vi "Init PWM Resources.vi"(8 "error in (no error)":errorcluster, 11 "Session in":refnum<class "Session.lvclass">) -> (0 "error out":errorcluster, 3 "Session out":refnum<class "Session.lvclass">)   [LabVIEW 2020, in "CTI.lvlib" / "Session.lvclass"]
uses:
  Session.lvclass
  GPIO Number.ctl
  PWM/PWM.lvclass
  Session.lvclass/Session.ctl
  CTI.lvlib
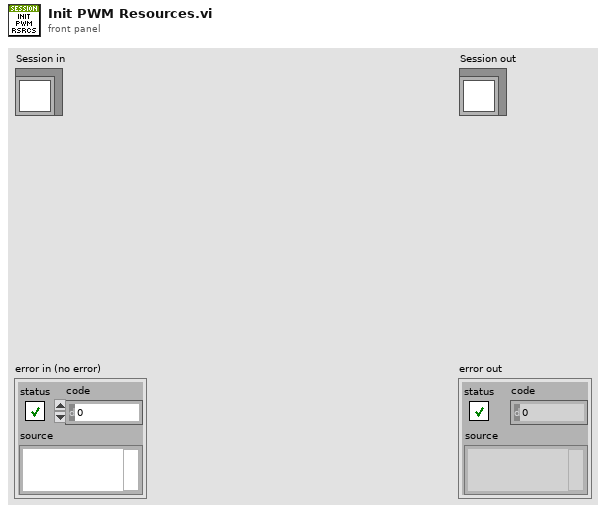
[diagram p1: front panel]
types:
  T1 = typedef "CTI.lvlib/GPIO Number.ctl" = i8
  T2 = typedef "CTI.lvlib/Session.lvclass/Resources.ctl" = cluster{"GPIO":map{T1, refnum<class "GPIO.lvclass">}, "AI":map{T3, refnum<class "AI.lvclass">}, "PWM":map{T1, refnum<class "PWM.lvclass">}, "UART":map{T4, refnum<class "UART.lvclass">}, "I2C":map{T5, refnum<class "I2C.lvclass">}, "SPI":map{T6, refnum<class "SPI.lvclass">}, "CS":map{T1, refnum<class "SPI CS.lvclass">}}
  T3 = typedef "CTI.lvlib/ADC Number.ctl" = i8
  T4 = typedef "CTI.lvlib/UART Number.ctl" = i8
  T5 = typedef "CTI.lvlib/I2C Number.ctl" = i8
  T6 = typedef "CTI.lvlib/SPI Number.ctl" = i8
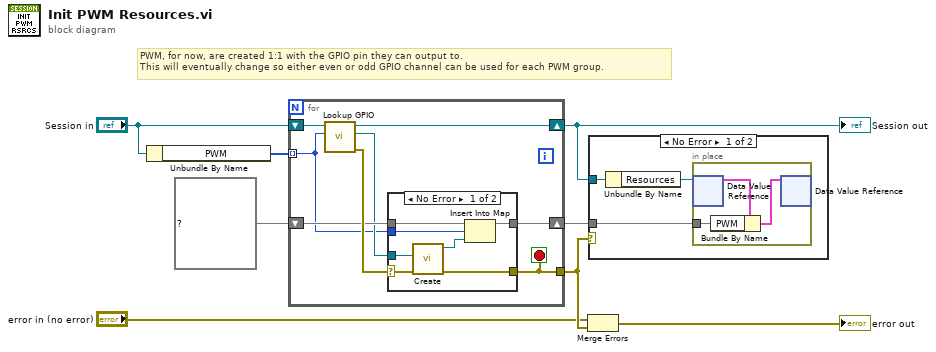
[diagram p0: block diagram]
diagram:
  # "PWM, for now, are created 1:1 with the GPIO pin they can output to.\nThis will eventually change so either even or odd GPIO channel can be used for each PWM group."
  n1 = Unbundle By Name("Session in") -> ("PWM"=w2:T1[])
  n2 = for {
    tunnel: w2 -> [w9] mode=indexing
    shift-right: [w14] -> w3
    shift-left: map{T1, refnum<class "PWM.lvclass">} {} ("PWM") -> [w15]
    shift-right: [w12] -> w8
    shift-left: "Session in" -> [w13]
    tunnel: [w10] -> w7
    stop <- w10 stop-if-true
    n3 = call "Lookup GPIO.vi"("GPIO #"=w9, "Session in"=w13) -> ("error out"=w16:errorcluster, "GPIO"=w11:refnum<class "GPIO.lvclass">, "Session out"=w12:refnum<class "Session.lvclass">)  [unwired: 7 in]
    n4 = case shown="No Error" w16 {
      selector: w16 -> [w19 w25]
      tunnel: w15 -> [w23 w24]
      tunnel: [w22 w24] -> w14
      tunnel: w11 -> [w20 _]
      tunnel: w9 -> [w21 _]
      tunnel: [w18 w25] -> w10
      frame No Error {
        n5 = call "Create.vi"("error in (no error)"=w19, "GPIO"=w20) -> ("error out"=w18:errorcluster, "PWM out"=w17:refnum<class "PWM.lvclass">)  [unwired: 8 in]
        n6 = Insert Into Map(map in=w23, key=w21, value=w17) -> (map out=w22:map{T1, refnum<class "PWM.lvclass">})  [unwired: 2 out]
      }
      frame Error {
      }
    }
  }
  "Session out" <- w8
  n7 = Merge Errors("error in (no error)", w7) -> (→"error out":errorcluster)
  n8 = case shown="No Error" w7 {
    tunnel: w3 -> [w26 _]
    tunnel: w8 -> [w28 _]
    frame No Error {
      n9 = Unbundle By Name(w28) -> ("Resources"=w27:refnum<data-value>)
      n10 = in-place {
        in-place-border: w26 -> [w30]
        n11 = in-place-dvr #1(w27) -> (w31:T2)  [unwired: 1 out]
        n12 = Bundle By Name(cluster=w31, "PWM"=w30) -> (w29:T2)
        n13 = in-place-dvr #1(w29) -> ()  [unwired: 2 out]
      }
    }
    frame Error {
    }
  }
